vi "GFL Config Parse.vi"(0 "Config File Path":path=path "C:/Automation/Configurations/VALEW.config", 11 "Error In":errorcluster) -> (4 "Pass/Fail?":bool, 6 "Report Text":string, 8 "GFL_config":T1, 15 "Error Out":errorcluster)   [LabVIEW 2016]
uses:
  type defs/GFL Config.ctl
  <vilib>/Utility/config.llb/Read Key (String).vi
  <vilib>/Utility/config.llb/Read Key (Boolean).vi
  <vilib>/Utility/config.llb/NI_LVConfig.lvlib
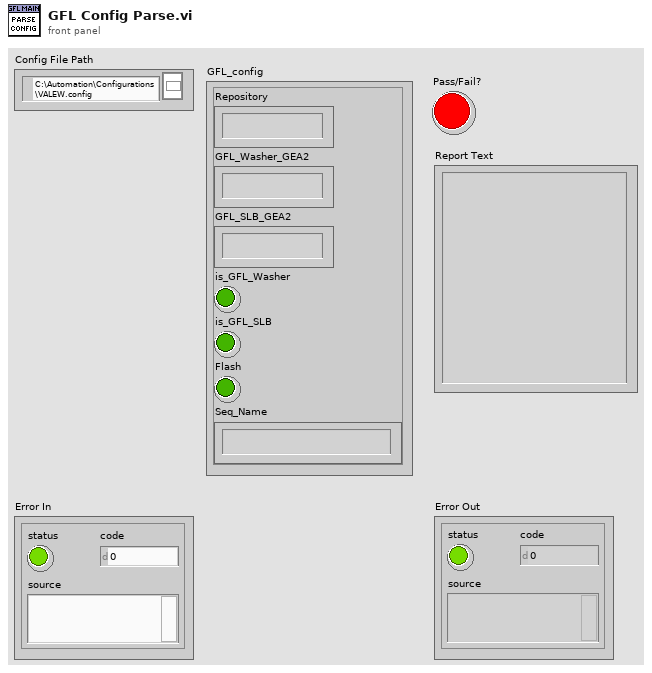
[diagram p1: front panel]
types:
  T1 = typedef "GFL Config.ctl" = cluster{"Repository":string, "GFL_Washer_GEA2":string, "GFL_SLB_GEA2":string, "is_GFL_Washer":bool, "is_GFL_SLB":bool, "Flash":bool, "Seq_Name":string}
  T2 = typedef "NI_LVConfig.lvlib/Config Data RefNum.ctl" = refnum<k1>
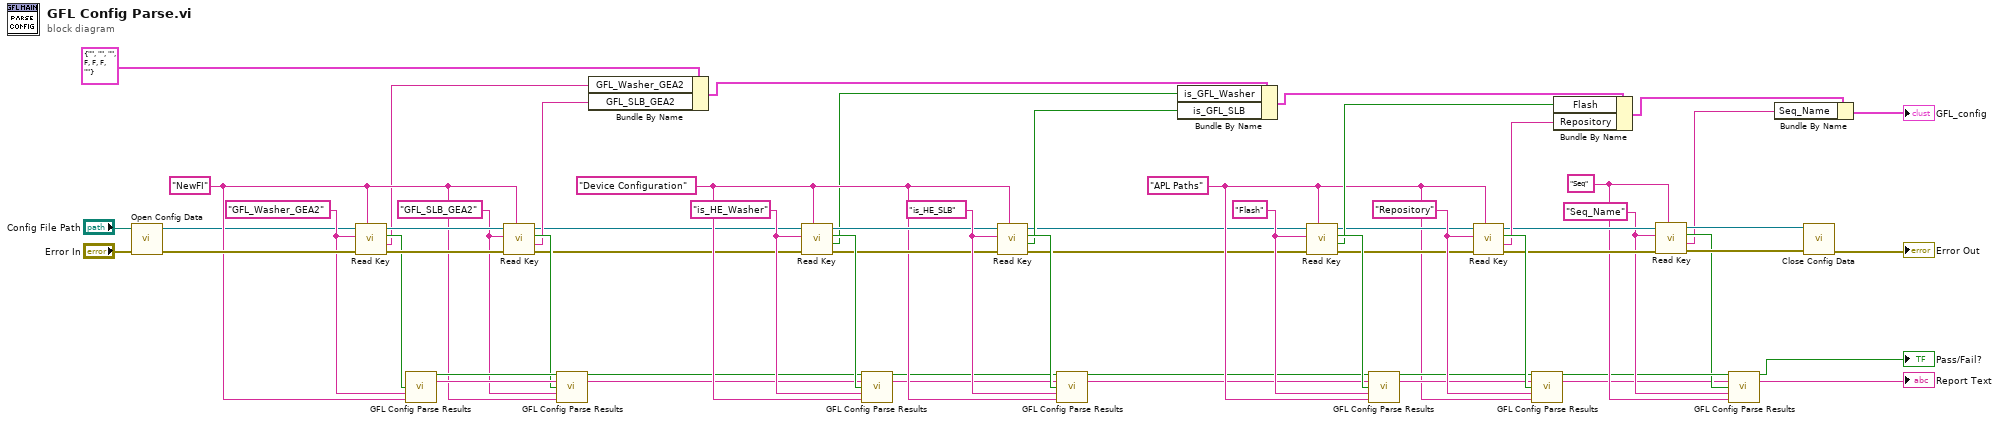
[diagram p0: block diagram]
diagram:
  w26 = "Seq_Name" ("key")
  w25 = "Seq" ("section")
  w38 = "Repository" ("key")
  w47 = "is_HE_SLB" ("key")
  w49 = "Flash" ("key")
  w22 = "APL Paths" ("section")
  w51 = "is_HE_Washer" ("key")
  w43 = "Device Configuration" ("section")
  w53 = "GFL_SLB_GEA2" ("key")
  w58 = "GFL_Washer_GEA2" ("key")
  w48 = "NewFI" ("section")
  n1 = call <vilib>:"Open Config Data.vi"("error in (no error)"="Error In", "configuration file path"="Config File Path") -> ("error out"=w61:errorcluster, "refnum"=w31:T2)  [unwired: 7 in, 1 out]
  n2 = call-poly <vilib>:"Read Key.vi"("section"=w48, "error in (no error)"=w61, "key"=w58, "refnum"=w31) -> ("error out"=w62:errorcluster, "value"=w13:string, "found?"=w57:bool, "refnum out"=w63:T2)  [unwired: 4 in]
  n3 = call "GFL Config Parse Results.vi"("found?"=w57, "key"=w58, "section"=w48) -> ("Pass/Fail"=w56:bool, "Report Text"=w55:string)  [unwired: 11 in]
  n4 = call-poly <vilib>:"Read Key.vi"("section"=w48, "error in (no error)"=w62, "key"=w53, "refnum"=w63) -> ("error out"=w7:errorcluster, "value"=w14:string, "found?"=w54:bool, "refnum out"=w8:T2)  [unwired: 4 in]
  n5 = call "GFL Config Parse Results.vi"("Previous Pass/Fail"=w56, "Previous Report Text"=w55, "found?"=w54, "key"=w53, "section"=w48) -> ("Pass/Fail"=w11:bool, "Report Text"=w12:string)  [unwired: 9 in]
  n6 = Bundle By Name(cluster=T1 {"Repository"="", "GFL_Washer_GEA2"="", "GFL_SLB_GEA2"="", "is_GFL_Washer"=FALSE, "is_GFL_SLB"=FALSE, "Flash"=FALSE, "Seq_Name"=""} ("VALEW_config"), "GFL_Washer_GEA2"=w13, "GFL_SLB_GEA2"=w14) -> (w10:T1)
  n7 = call-poly <vilib>:"Read Key.vi"("section"=w43, "error in (no error)"=w7, "key"=w51, "refnum"=w8) -> ("error out"=w44:errorcluster, "value"=w9:bool, "found?"=w52:bool, "refnum out"=w45:T2)  [unwired: 4 in]
  n8 = call "GFL Config Parse Results.vi"("Previous Pass/Fail"=w11, "Previous Report Text"=w12, "found?"=w52, "key"=w51, "section"=w43) -> ("Pass/Fail"=w42:bool, "Report Text"=w41:string)  [unwired: 9 in]
  n9 = call-poly <vilib>:"Read Key.vi"("section"=w43, "error in (no error)"=w44, "key"=w47, "refnum"=w45) -> ("error out"=w4:errorcluster, "value"=w6:bool, "found?"=w46:bool, "refnum out"=w5:T2)  [unwired: 4 in]
  n10 = call "GFL Config Parse Results.vi"("Previous Pass/Fail"=w42, "Previous Report Text"=w41, "found?"=w46, "key"=w47, "section"=w43) -> ("Pass/Fail"=w3:bool, "Report Text"=w2:string)  [unwired: 9 in]
  n11 = Bundle By Name(cluster=w10, "is_GFL_Washer"=w9, "is_GFL_SLB"=w6) -> (w1:T1)
  n12 = call-poly <vilib>:"Read Key.vi"("section"=w22, "error in (no error)"=w4, "key"=w49, "refnum"=w5) -> ("error out"=w33:errorcluster, "value"=w40:bool, "found?"=w50:bool, "refnum out"=w34:T2)  [unwired: 4 in]
  n13 = call "GFL Config Parse Results.vi"("Previous Pass/Fail"=w3, "Previous Report Text"=w2, "found?"=w50, "key"=w49, "section"=w22) -> ("Pass/Fail"=w36:bool, "Report Text"=w35:string)  [unwired: 9 in]
  n14 = call-poly <vilib>:"Read Key.vi"("section"=w22, "error in (no error)"=w33, "key"=w38, "refnum"=w34) -> ("error out"=w30:errorcluster, "value"=w32:string, "found?"=w39:bool, "refnum out"=w28:T2)  [unwired: 4 in]
  n15 = call "GFL Config Parse Results.vi"("Previous Pass/Fail"=w36, "Previous Report Text"=w35, "found?"=w39, "key"=w38, "section"=w22) -> ("Pass/Fail"=w24:bool, "Report Text"=w16:string)  [unwired: 9 in]
  n16 = Bundle By Name(cluster=w1, "Flash"=w40, "Repository"=w32) -> (w21:T1)
  n17 = call-poly <vilib>:"Read Key.vi"("section"=w25, "error in (no error)"=w30, "key"=w26, "refnum"=w28) -> ("error out"=w29:errorcluster, "value"=w20:string, "found?"=w23:bool, "refnum out"=w27:T2)  [unwired: 4 in]
  n18 = call "GFL Config Parse Results.vi"("Previous Pass/Fail"=w24, "Previous Report Text"=w16, "found?"=w23, "key"=w26, "section"=w25) -> ("Pass/Fail"=→"Pass/Fail?":bool, "Report Text"=→"Report Text":string)  [unwired: 9 in]
  n19 = Bundle By Name(cluster=w21, "Seq_Name"=w20) -> (→"GFL_config":T1)
  n20 = call <vilib>:"Close Config Data.vi"("error in (no error)"=w29, "refnum"=w27) -> ("error out"=→"Error Out":errorcluster)  [unwired: 8 in, 1 out]
